vi "Calculate Common Root.vi"(8 "error in (no error)":errorcluster, 10 "Generated Files":path[](array[path])) -> (0 "error out":errorcluster, 2 "Root Path":path)   [LabVIEW 2014, in "G CLI LvBuild.lvlib"]
uses:
  G CLI LvBuild.lvlib
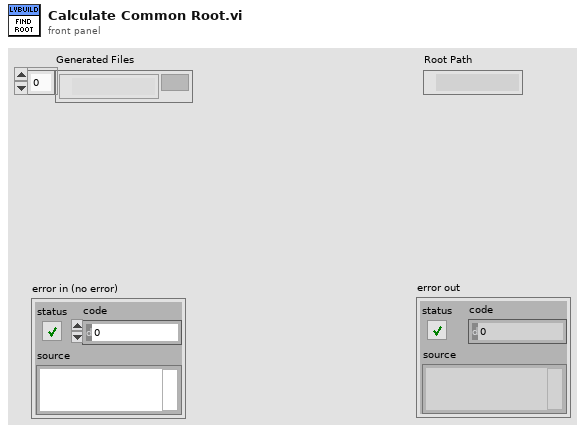
[diagram p1: front panel]
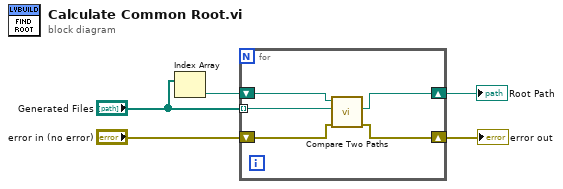
[diagram p0: block diagram]
diagram:
  n1 = Index Array(array="Generated Files") -> (element=w4:path)  [unwired: 1 in]
  n2 = for {
    tunnel: "Generated Files" -> [w10] mode=indexing
    shift-right: [w8] -> w3
    shift-left: w4 -> [w9]
    shift-right: [w6] -> w1
    shift-left: "error in (no error)" -> [w7]
    n3 = call <vilib>:"Compare Two Paths.vi"("error in (no error)"=w7, "Path 2"=w10, "Path 1"=w9) -> ("error out"=w6:errorcluster, "Common Path"=w8:path)  [unwired: 5 in, 2 out]
  }
  "Root Path" <- w3
  "error out" <- w1
